vi "Actor Core.vi"(8 "error in":errorcluster, 11 "Nested in":refnum<class "UI Actor.lvclass">) -> (0 "error out":errorcluster, 3 "Actor out":refnum<class "Actor.lvclass">)   [LabVIEW 2020, in "UI Actor.lvlib" / "UI Actor.lvclass"]
doc: "(<B>Filename</B>: Actor Framework.lvlib:Actor.lvclass:Actor Core.vi)\n\nReceives messages to the actor, reacts to them, and initiates any error handling that may shut the actor down.\n\nDescendant classes may override this VI to append parallel tasks for the actor to complete while it handles messages. Overrides use the Call Parent Method node."
uses:
  UI Actor.lvclass
  C:/Program Files (x86)/National Instruments/LabVIEW 2020/vi.lib/ActorFramework/Actor/Actor.lvclass
  <vilib>/ActorFramework/Actor/Actor.lvclass
  <vilib>/ActorFramework/Actor/Actor.lvclass/Actor.ctl
  <vilib>/ActorFramework/Message Enqueuer/Message Enqueuer.lvclass/Message Enqueuer.ctl
  UI Actor.lvclass/UI Actor.ctl
  <vilib>/ActorFramework/Message Enqueuer/Init from Existing Queue.vi
  <vilib>/ActorFramework/Message Enqueuer/Enqueue.vi
  <vilib>/ActorFramework/Stop Msg/Stop Msg.lvclass
  C:/Program Files (x86)/National Instruments/LabVIEW 2020/vi.lib/ActorFramework/Message/Message.lvclass
  <vilib>/ActorFramework/Message Priority Queue/Priority Enqueue.vi
  <vilib>/ActorFramework/Message Enqueuer/Message Enqueuer.lvclass
  Abstract/Serial Device/Serial Device.lvclass
panel:
  in  "READ PIN":bool
  out "Pin Response":bool
  in  "Pin[I]":dbl
  in  "WRITE PIN":bool
  in  "Pin[P]":dbl
  in  "1/0":bool
  in  "READ PORT":bool
  in  "Port[R]":dbl
  out "Binary Number":T1
  in  "SEND ADC":bool
  in  "Channel":enum16{"2", "1"}(ring)
  out "Response[A]":i32(slide) scale=0.0..100.0
  in  "WRITE PORT":bool
  out "GENERAL RESPONSE [R]":string
  in  "Port[W]":dbl
  in  "Binary Number":T2
  # "READ PIN"
  # "WRITE PIN"
  # "READ PORT"
  # "SEND ADC"
  # "Simulated Device"
  # "WRITE PORT"
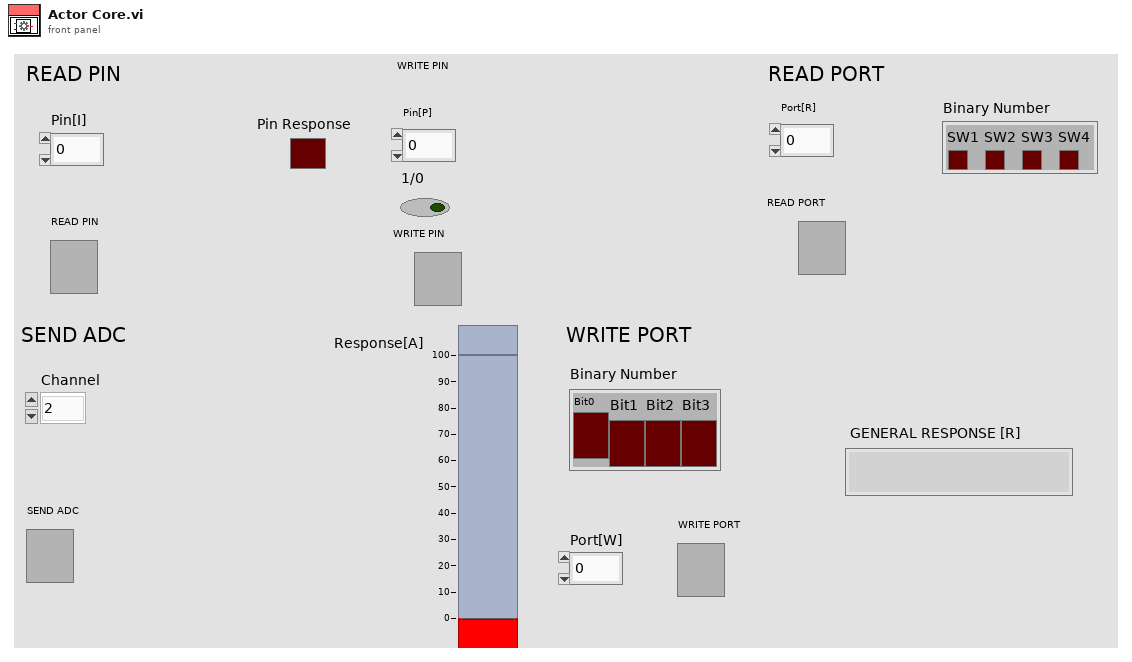
[diagram p1: front panel]
types:
  T1 = cluster{"SW1":bool, "SW2":bool, "SW3":bool, "SW4":bool, "[4]":bool, "[5]":bool, "[6]":bool, "[7]":bool, "[8]":bool}
  T2 = cluster{"Bit0":bool, "Bit1":bool, "Bit2":bool, "Bit3":bool}
  T3 = cluster{"Stop":refnum<user-event>, "Waveform Graph":refnum<user-event>, "Binary Number":refnum<user-event>, " Response[R] ":refnum<user-event>, "Pin":refnum<user-event>, "Response[A]":refnum<user-event>}
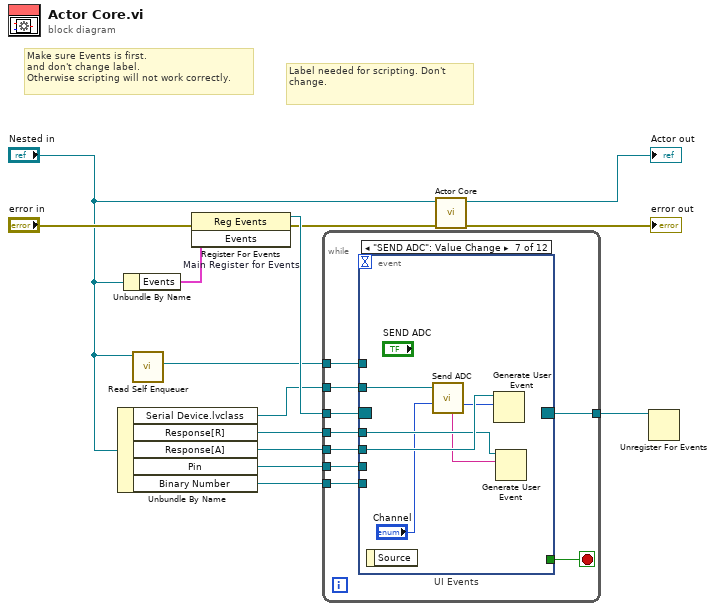
[diagram p0: block diagram]
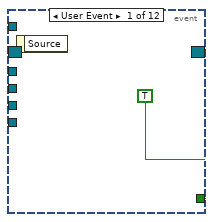
[diagram p2: hidden frame]
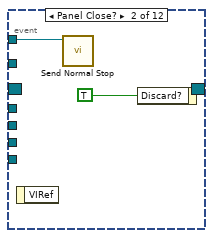
[diagram p3: hidden frame]
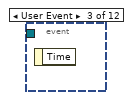
[diagram p4: hidden frame]
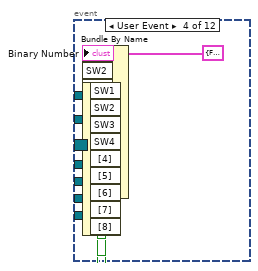
[diagram p5: hidden frame]
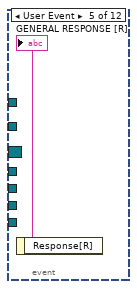
[diagram p6: hidden frame]
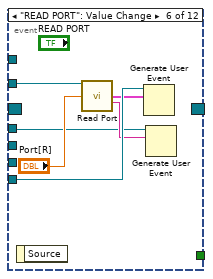
[diagram p7: hidden frame]
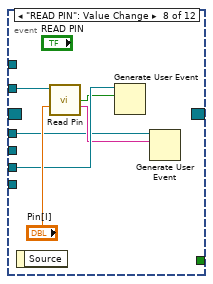
[diagram p8: hidden frame]
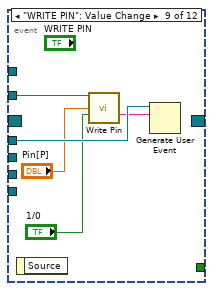
[diagram p9: hidden frame]
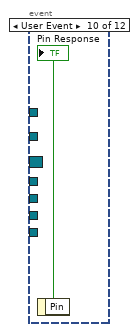
[diagram p10: hidden frame]
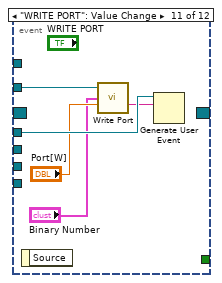
[diagram p11: hidden frame]
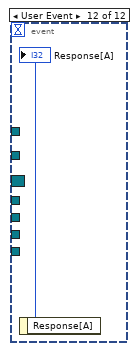
[diagram p12: hidden frame]
diagram:
  # "Label needed for scripting. Don't change."
  # "Make sure Events is first.\nand don't change label.\nOtherwise scripting will not work correctly."
  n1 = Unbundle By Name("Nested in") -> ("Serial Device.lvclass"=w5:refnum<class "Serial Device.lvclass">, "Response[R]"=w4:refnum<user-event>, "Response[A]"=w3:refnum<user-event>, "Pin"=w2:refnum<user-event>, "Binary Number"=w1:refnum<user-event>)
  n2 = Unbundle By Name("Nested in") -> ("Events"=w11:T3)
  n3 = call <vilib>:"Read Self Enqueuer.vi"("Actor"="Nested in") -> ("Self Enqueuer"=w9:refnum<class "Message Enqueuer.lvclass">)  [unwired: 10 in]
  n4 = register-events "Main Register for Events"(error in="error in", w11) -> (reference out=w12:refnum<event-registration>, error out=w7:errorcluster)  [unwired: 1 in]
  n5 = while {
    tunnel: w12 -> [w23]
    tunnel: [w21] -> w10
    tunnel: w9 -> [w20]
    tunnel: w5 -> [w19]
    tunnel: w4 -> [w18]
    tunnel: w3 -> [w17]
    tunnel: w2 -> [w16]
    tunnel: w1 -> [w15]
    stop <- w22 stop-if-true
    n6 = event "UI Events" shown="[6] \"SEND ADC\": Value Change" {
      selector: w23 -> [_ _ _ _ _ _ _ _ _ _ _ _]
      dyn-events: [_ _ _ _ _ _ _ _ _ _ _ _] -> w21
      timeout: _ -> [_ _ _ _ _ _ _ _ _ _ _ _]
      tunnel: [TRUE _ _ _ _ _ _ _ _ _ _ _] -> w22
      tunnel: w20 -> [_ w25 _ _ _ _ _ _ _ _ _ _]
      tunnel: w19 -> [_ _ _ _ _ w44 w48 w56 w61 _ w66 _]
      tunnel: w18 -> [_ _ _ _ _ w39 w49 w51 w60 _ w67 _]
      tunnel: w17 -> [_ _ _ _ _ _ w50 _ _ _ _ _]
      tunnel: w16 -> [_ _ _ _ _ _ _ w54 _ _ _ _]
      tunnel: w15 -> [_ _ _ _ _ w43 _ _ _ _ _ _]
      event User Event {
        n7 = event-data() -> ()  [unwired: 1 in, 1 out]
      }
      event Panel Close? {
        n8 = event-data() -> ()  [unwired: 1 in, 1 out]
        n9 = call <vilib>:"Send Normal Stop.vi"("Message Enqueuer"=w25) -> ()  [unwired: 10 in, 1 out]
        n10 = event-data("Discard?"=TRUE) -> ()  [unwired: 1 in, 1 out]
      }
      event User Event {
        n11 = event-data() -> ()  [unwired: 1 in, 1 out]
      }
      event User Event {
        n12 = event-data() -> ("SW1"=w35:bool, "SW2"=w34:bool, "SW3"=w33:bool, "SW4"=w32:bool, "[4]"=w31:bool, "[5]"=w30:bool, "[6]"=w29:bool, "[7]"=w28:bool, "[8]"=w27:bool)  [unwired: 1 in]
        n13 = Bundle By Name(cluster=T1 {"SW1"=FALSE, "SW2"=FALSE, "SW3"=FALSE, "SW4"=FALSE, "[4]"=FALSE, "[5]"=FALSE, "[6]"=FALSE, "[7]"=FALSE, "[8]"=FALSE} ("Binary Number"), "SW1"=w35, "SW2"=w34, "SW3"=w33, "SW4"=w32, "[4]"=w31, "[5]"=w30, "[6]"=w29, "[7]"=w28, "[8]"=w27) -> (→"Binary Number":T1)
      }
      event User Event {
        n14 = event-data() -> ("Response[R]"=→"GENERAL RESPONSE [R]":string)  [unwired: 1 in]
      }
      event "READ PORT": Value Change {
        n15 = event-data() -> ()  [unwired: 1 in, 1 out]
        n16 = call-dynamic "Read Port.vi"("Serial Device in"=w44, "Port"="Port[R]") -> ("Binary Number"=w42:T1, "Response"=w40:string)  [unwired: 9 in, 3 out]
        n17 = Generate User Event(user event=w43, event data cluster=w42) -> ()  [unwired: 2 in, 2 out]
        n18 = Generate User Event(user event=w39, event data cluster=w40) -> ()  [unwired: 2 in, 2 out]
      }
      event "SEND ADC": Value Change {
        n19 = event-data() -> ()  [unwired: 1 in, 1 out]
        n20 = call-dynamic "Send ADC.vi"("Serial Device in"=w48, "Channel"="Channel") -> ("Response"=w45:i32, "command"=w46:string)  [unwired: 9 in, 3 out]
        n21 = Generate User Event(user event=w50, event data cluster=w45) -> ()  [unwired: 2 in, 2 out]
        n22 = Generate User Event(user event=w49, event data cluster=w46) -> ()  [unwired: 2 in, 2 out]
      }
      event "READ PIN": Value Change {
        n23 = event-data() -> ()  [unwired: 1 in, 1 out]
        n24 = call-dynamic "Read Pin.vi"("Serial Device in"=w56, "Port"="Pin[I]") -> ("Pin"=w53:bool, "Response"=w52:string)  [unwired: 9 in, 3 out]
        n25 = Generate User Event(user event=w54, event data cluster=w53) -> ()  [unwired: 2 in, 2 out]
        n26 = Generate User Event(user event=w51, event data cluster=w52) -> ()  [unwired: 2 in, 2 out]
      }
      event "WRITE PIN": Value Change {
        n27 = event-data() -> ()  [unwired: 1 in, 1 out]
        n28 = call-dynamic "Write Pin.vi"("Serial Device in"=w61, "Pin"="Pin[P]", "1/0"="1/0") -> ("Read"=w59:string)  [unwired: 9 in, 3 out]
        n29 = Generate User Event(user event=w60, event data cluster=w59) -> ()  [unwired: 2 in, 2 out]
      }
      event User Event {
        n30 = event-data() -> ("Pin"=→"Pin Response":bool)  [unwired: 1 in]
      }
      event "WRITE PORT": Value Change {
        n31 = event-data() -> ()  [unwired: 1 in, 1 out]
        n32 = call-dynamic "Write Port.vi"("Serial Device in"=w66, "Binary Number"="Binary Number", "Port 2"="Port[W]") -> ("Response"=w65:string)  [unwired: 9 in, 3 out]
        n33 = Generate User Event(user event=w67, event data cluster=w65) -> ()  [unwired: 2 in, 2 out]
      }
      event User Event {
        n34 = event-data() -> ("Response[A]"=→"Response[A]":i32)  [unwired: 1 in]
      }
    }
  }
  n35 = call-parent "Actor Core.vi"("error in"=w7, "Actor in"="Nested in") -> ("error out"=→"error out":errorcluster, "Actor out"=→"Actor out":refnum<class "Actor.lvclass">)  [unwired: 8 in]
  n36 = Unregister For Events(event registration refnum=w10) -> ()  [unwired: 1 in, 1 out]
